vi "NIIE_Export_Clipboard.vi"(7 "Is Copy? (F)":bool, 8 "error in (no error)":errorcluster, 11 "Data in":T1={"Class"={"Ants"=refnum, "Layer"=refnum, "Templates"=refnum, "Icon"=refnum, "Glyph"=refnum, "Settings"=refnum, "Tools"=refnum}, "Ref"={"Add Layer"=refnum, "Remove Layer"=refnum, "Line Text"=[], "Body Text Spec"=refnum, "DNL_Font"=refnum, "glyph path str"=refnum, "templates path str"=refnum, "Arrow Up"=refnum, "Arrow Down"=refnum, "IE VI Ref"=refnum, "Glyphs tree"=refnum, "Templates tree"=refnum, "Layer Icon Text"=refnum, "Layer Template"=refnum, "Clipboard"=refnum, "BW icon in"=refnum, "Color icon in"=refnum, "Layer Clust"=refnum, "Body Text"=refnum, "DNL_Framework Templates"=refnum, "Search Templates"=refnum, "TextMarker"=refnum, "Tab Control"=refnum, "Search Glyphs"=refnum, "Line Color"=refnum, "DNL_Glyphs []"=refnum, "Fill Color"=refnum, "Tools"=refnum, "Glyphs tree"=refnum, "Icon"=refnum, "Preview"=refnum, "Ants"=refnum, "Terminals"=refnum, "menu reference"=refnum, "LayerNames"=[], "GlyphLoadAnimation"=refnum, "TemplateLoadAnimation"=refnum, "refreshGlyphs"=refnum, "refreshTemplates"=refnum}, "Support"={"AntsRect"={"left"=0, "top"=0, "right"=0, "bottom"=0}, "Mouse Move Coords"={"Horizontal"=0, "Vertical"=0}, "Mouse Down Coords"={"Horizontal"=0, "Vertical"=0}, "Temp Coord"={"Horizontal"=0, "Vertical"=0}, "Action"=enum."Default", "Edge Color"=4914962, "Fill Color"=16860, "Mouse Down?"=FALSE, "Draft Mode?"=FALSE, "Temp Icon"=bytes[3102], "CTRL Pressed"=FALSE, "Move Selection?"=FALSE, "AntsRect Orig"={"left"=0, "top"=0, "right"=0, "bottom"=0}, "Text"="", "TM Set?"=FALSE, "Mouse inside icon?"=FALSE, "Tool (old value)"=0, "Pencil Move Color"=0, "Swap Colors?"=FALSE, "Shift pressed?"=FALSE}}) -> (0 "error out":errorcluster, 3 "Data out":T1={"Class"={"Ants"=refnum, "Layer"=refnum, "Templates"=refnum, "Icon"=refnum, "Glyph"=refnum, "Settings"=refnum, "Tools"=refnum}, "Ref"={"Add Layer"=refnum, "Remove Layer"=refnum, "Line Text"=[], "Body Text Spec"=refnum, "DNL_Font"=refnum, "glyph path str"=refnum, "templates path str"=refnum, "Arrow Up"=refnum, "Arrow Down"=refnum, "IE VI Ref"=refnum, "Glyphs tree"=refnum, "Templates tree"=refnum, "Layer Icon Text"=refnum, "Layer Template"=refnum, "Clipboard"=refnum, "BW icon in"=refnum, "Color icon in"=refnum, "Layer Clust"=refnum, "Body Text"=refnum, "DNL_Framework Templates"=refnum, "Search Templates"=refnum, "TextMarker"=refnum, "Tab Control"=refnum, "Search Glyphs"=refnum, "Line Color"=refnum, "DNL_Glyphs []"=refnum, "Fill Color"=refnum, "Tools"=refnum, "Glyphs tree"=refnum, "Icon"=refnum, "Preview"=refnum, "Ants"=refnum, "Terminals"=refnum, "menu reference"=refnum, "LayerNames"=[], "GlyphLoadAnimation"=refnum, "TemplateLoadAnimation"=refnum, "refreshGlyphs"=refnum, "refreshTemplates"=refnum}, "Support"={"AntsRect"={"left"=0, "top"=0, "right"=0, "bottom"=0}, "Mouse Move Coords"={"Horizontal"=0, "Vertical"=0}, "Mouse Down Coords"={"Horizontal"=0, "Vertical"=0}, "Temp Coord"={"Horizontal"=0, "Vertical"=0}, "Action"=enum."Default", "Edge Color"=4914962, "Fill Color"=16860, "Mouse Down?"=FALSE, "Draft Mode?"=FALSE, "Temp Icon"=bytes[3102], "CTRL Pressed"=FALSE, "Move Selection?"=FALSE, "AntsRect Orig"={"left"=0, "top"=0, "right"=0, "bottom"=0}, "Text"="", "TM Set?"=FALSE, "Mouse inside icon?"=FALSE, "Tool (old value)"=0, "Pencil Move Color"=0, "Swap Colors?"=FALSE, "Shift pressed?"=FALSE}})   [LabVIEW 2021]
uses:
  Controls/IE Data.ctl
  Class/Ants/Ants.lvclass
  Class/FakedArray/FakedArray.lvclass
  Class/Icon Library/Glyph.lvclass
  Class/Settings/Settings.lvclass
  Class/Tools/Tools Paint.lvclass
  vi.lib/LabVIEW Icon API/lv_icon/Classes/Icon/Icon.lvclass
  Controls/IE Classes.ctl
  Controls/References Cluster.ctl
  Controls/SupportClass.ctl
  <vilib>/Utility/miscctls.llb/LVPoint32TypeDef.ctl
  Controls/ENUM_SupportClass_Action.ctl
  vi.lib/LabVIEW Icon API/lv_icon/Controls/IEColor.ctl
  vi.lib/LabVIEW Icon API/lv_icon/Classes/Icon Framework/Icon Framework.lvclass
  C:/Users/Mark.Balla/Projects/MB Tools/ICON Editor LV/labview-icon-editor-main LV2021 2024-10-24/vi.lib/LabVIEW Icon API/lv_icon/Classes/Layer/Layer.lvclass
  vi.lib/LabVIEW Icon API/lv_icon/lv_icon.lvlib
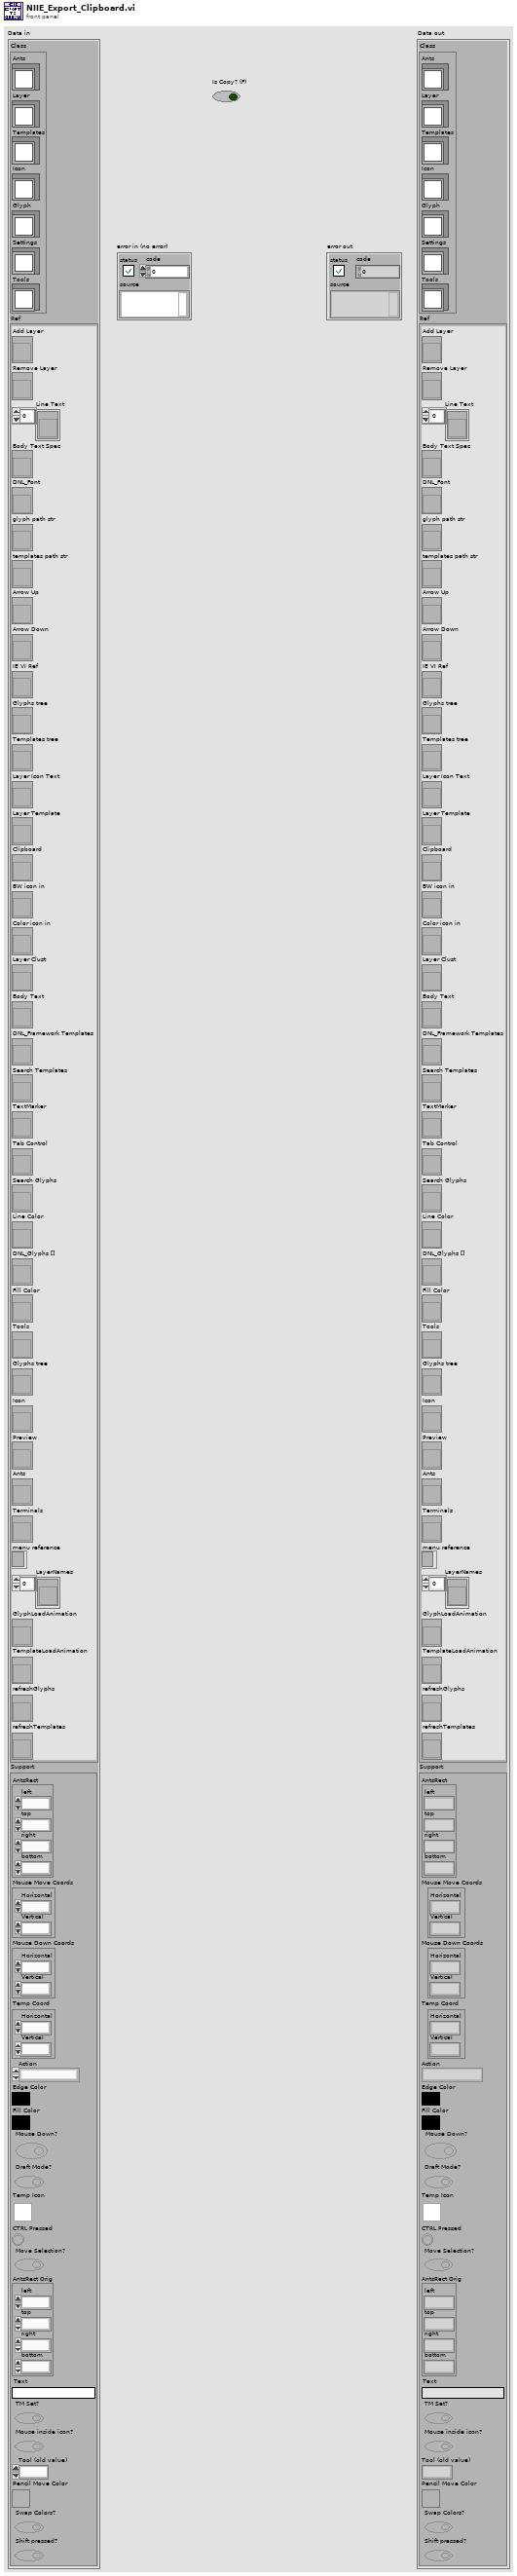
[diagram p1: front panel]
types:
  T1 = typedef "IE Data.ctl" = cluster{"Class":T2, "Ref":T3, "Support":T4}
  T2 = typedef "IE Classes.ctl" = cluster{"Ants":refnum<class "Ants.lvclass">, "Layer":refnum<class "FakedArray.lvclass">, "Templates":refnum<class "FakedArray.lvclass">, "Icon":refnum<class "Icon.lvclass">, "Glyph":refnum<class "Glyph.lvclass">, "Settings":refnum<class "Settings.lvclass">, "Tools":refnum<class "Tools Paint.lvclass">}
  T3 = typedef "References Cluster.ctl" = cluster{"Add Layer":refnum<vi>, "Remove Layer":refnum<vi>, "Line Text":refnum<vi>[], "Body Text Spec":refnum<vi>, "DNL_Font":refnum<vi>, "glyph path str":refnum<vi>, "templates path str":refnum<vi>, "Arrow Up":refnum<vi>, "Arrow Down":refnum<vi>, "IE VI Ref":refnum<vi>, "Glyphs tree":refnum<vi>, "Templates tree":refnum<vi>, "Layer Icon Text":refnum<vi>, "Layer Template":refnum<vi>, "Clipboard":refnum<vi>, "BW icon in":refnum<vi>, "Color icon in":refnum<vi>, "Layer Clust":refnum<vi>, "Body Text":refnum<vi>, "DNL_Framework Templates":refnum<vi>, "Search Templates":refnum<vi>, "TextMarker":refnum<vi>, "Tab Control":refnum<vi>, "Search Glyphs":refnum<vi>, "Line Color":refnum<vi>, "DNL_Glyphs []":refnum<vi>, "Fill Color":refnum<vi>, "Tools":refnum<vi>, "Glyphs tree":refnum<vi>, "Icon":refnum<vi>, "Preview":refnum<vi>, "Ants":refnum<vi>, "Terminals":refnum<vi>, "menu reference":refnum<k9>, "LayerNames":refnum<vi>[], "GlyphLoadAnimation":refnum<vi>, "TemplateLoadAnimation":refnum<vi>, "refreshGlyphs":refnum<vi>, "refreshTemplates":refnum<vi>}
  T4 = typedef "SupportClass.ctl" = cluster{"AntsRect":cluster{"left":i16, "top":i16, "right":i16, "bottom":i16}, "Mouse Move Coords":T5, "Mouse Down Coords":T5, "Temp Coord":T5, "Action":T6, "Edge Color":T7, "Fill Color":T7, "Mouse Down?":bool, "Draft Mode?":bool, "Temp Icon":picture, "CTRL Pressed":bool, "Move Selection?":bool, "AntsRect Orig":cluster{"left":i16, "top":i16, "right":i16, "bottom":i16}, "Text":string, "TM Set?":bool, "Mouse inside icon?":bool, "Tool (old value)":u32, "Pencil Move Color":u32, "Swap Colors?":bool, "Shift pressed?":bool}
  T5 = typedef "LVPoint32TypeDef.ctl" = cluster{"Horizontal":i32, "Vertical":i32}
  T6 = typedef "ENUM_SupportClass_Action.ctl" = enum16{"Default", "Move Selection", "Glyph Library", "Tool"}
  T7 = typedef "IEColor.ctl" = u32
  T8 = cluster{"left":i16, "top":i16, "right":i16, "bottom":i16}
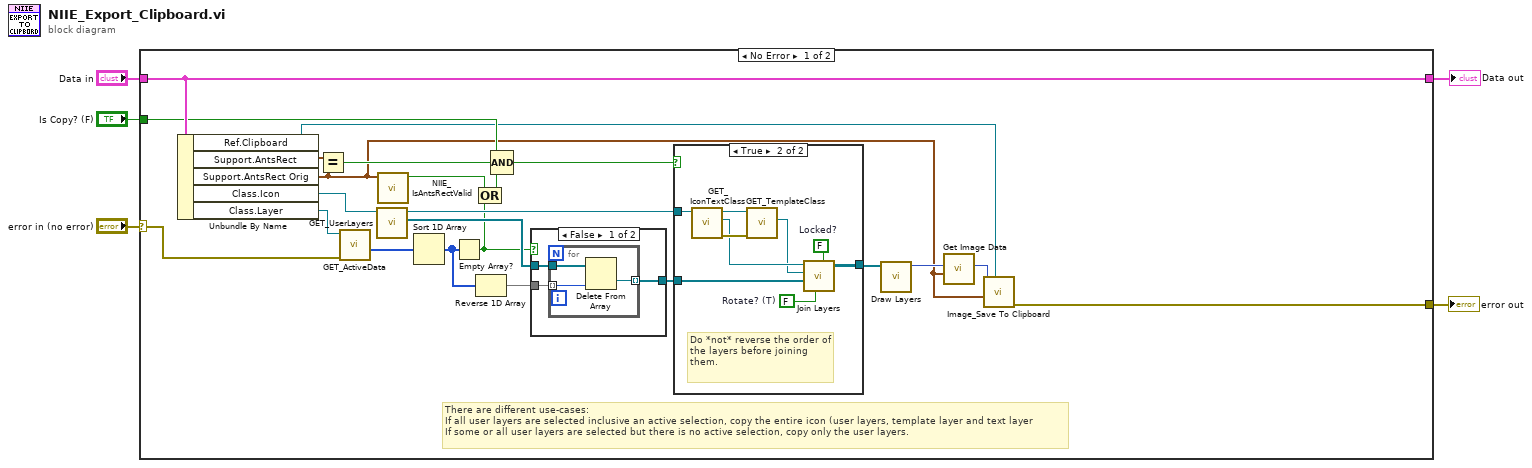
[diagram p0: block diagram]
diagram:
  n1 = case shown="No Error" "error in (no error)" {
    selector: "error in (no error)" -> [w27 w47]
    tunnel: [w28 w47] -> w4
    tunnel: [w18 w46] -> w3
    tunnel: "Data in" -> [w18 w46]
    tunnel: "Is Copy? (F)" -> [w9 _]
    frame No Error {
      # "There are different use-cases:\nIf all user layers are selected inclusive an active selection, copy the entire icon (user layers, template layer and text layer\nIf some or all user layers are selected but there is no active selection, copy only the user layers."
      n2 = Unbundle By Name(w18) -> ("Ref.Clipboard"=w8:refnum<vi>, "Support.AntsRect"=w11:T8, "Support.AntsRect Orig"=w6:T8, "Class.Icon"=w16:refnum<class "Icon.lvclass">, "Class.Layer"=w17:refnum<class "FakedArray.lvclass">)
      n3 = Equal?(x=w11, y=w6) -> (x = y?=w13:bool)
      n4 = call-dynamic "GET_ActiveData.vi"("Error"=w27, "FakedArray"=w17) -> ("Active Data [] Out"=w24:i32[])  [unwired: 9 out]
      n5 = call-dynamic "GET_UserLayers.vi"("Icon.lvclass in"=w16) -> ("All Layers"=w25:refnum<class "Layer.lvclass">[], "Icon.lvclass out"=w21:refnum<class "Icon.lvclass">)  [unwired: 1 in, 8 out]
      n6 = call "NIIE_IsAntsRectValid.vi"("Image Range"=w6) -> ("Valid? Out"=w19:bool)  [unwired: 10 out]
      n7 = Sort 1D Array(array=w24) -> (sorted array=w23:i32[])
      n8 = Empty Array?(array=w23) -> (empty?=w10:bool)
      n9 = Reverse 1D Array(array=w23) -> (reversed array=w22:i32[])
      n10 = Compound Arithmetic op=OR(w19, w10) -> (w14:bool)
      n11 = Compound Arithmetic op=AND(w9, w13, w14) -> (w12:bool)
      n12 = case shown="False" w10 {
        tunnel: w25 -> [w41 w45]
        tunnel: [w40 w45] -> w20
        tunnel: w22 -> [w39 _]
        frame False {
          n13 = for {
            tunnel: w41 -> [w43]
            tunnel: w39 -> [w44] mode=indexing
            tunnel: [w42] -> w40 mode=indexing
            n14 = Delete From Array(array=w43, index=w44) -> (deleted portion=w42:refnum<class "Layer.lvclass">)  [unwired: 1 in, 1 out]
          }
        }
        frame True {
        }
      }
      n15 = case shown="True" w12 {
        tunnel: w21 -> [_ w36]
        tunnel: [w29 w35] -> w15
        tunnel: w20 -> [w29 w32]
        frame False {
        }
        frame True {
          w30 = FALSE  # Locked?
          w31 = FALSE  # Rotate? (T)
          # "Do *not* reverse the order of the layers before joining them."
          n16 = call-dynamic "GET_IconTextClass.vi"("Icon.lvclass in"=w36) -> ("error out"=w38:errorcluster, "Icon Framework.lvclass"=w34:refnum<class "Icon Framework.lvclass">, "Icon.lvclass out"=w37:refnum<class "Icon.lvclass">)  [unwired: 1 in, 7 out]
          n17 = call-dynamic "GET_TemplateClass.vi"("error in (no error)"=w38, "Icon.lvclass in"=w37) -> ("Icon Framework.lvclass"=w33:refnum<class "Icon Framework.lvclass">)  [unwired: 9 out]
          n18 = call "Join Layers.vi"("Locked?"=w30, "Rotate? (T)"=w31, "User Layers"=w32, "Template"=w33, "Icon Text"=w34) -> ("Layer Out"=w35:refnum<class "Layer.lvclass">[])  [unwired: 1 in, 5 out]
        }
      }
      n19 = call "Draw Layers.vi"("Layers"=w15) -> ("Picture"=w26:picture)  [unwired: 4 in, 6 out]
      n20 = call "Get Image Data.vi"("Image Range"=w6, "Pic"=w26) -> ("Pic Out"=w7:picture)  [unwired: 1 in, 8 out]
      n21 = call "Image_Save To Clipboard.vi"("Image Ref"=w8, "Image Range"=w6, "Image"=w7) -> ("Error Out"=w28:errorcluster)  [unwired: 8 in]
    }
    frame Error {
    }
  }
  "error out" <- w4
  "Data out" <- w3
